vi "updated_hai-1.vi"() -> ()   [LabVIEW 2023]
uses:
  <vilib>/Utility/NIReport.llb/Report Type.ctl
  <vilib>/Utility/NIReport.llb/Append Text Table to Report (wrap).vi
  <vilib>/Utility/NIReport.llb/NI_report.lvclass
  <vilib>/Utility/NIReport.llb/NI_ReportGenerationCore.lvlib
  <vilib>/Utility/NIReport.llb/Excel/NI_Excel.lvclass
panel:
  out "Remaining_hours(hrs)":dbl
  out "Current flow out rate":dbl
  out "Current flow in rate":dbl
  out "Current water level  in litres:":dbl
  in  "Flow out rate(litres/sec)":dbl(slide) scale=0.0..10.0
  in  "Flow in rate(liters/sec)":dbl(slide) step=1.0 scale=0.0..10.0
  out "Water level is low":bool
  out "Water level is high":bool
  out "Tank":dbl(slide) scale=0.0..100.0
  in  "stop":bool
  in  "report file path":path
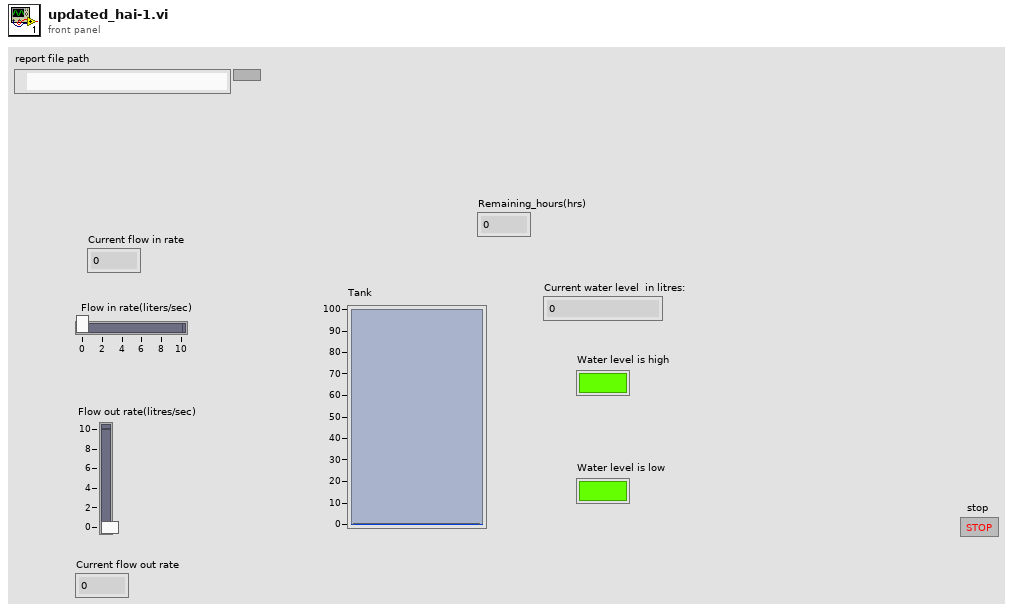
[diagram p1: front panel]
types:
  T1 = typedef "NI_ReportGenerationCore.lvlib/Report Type.ctl" = enum16{"HTML", "Word", "Excel"}
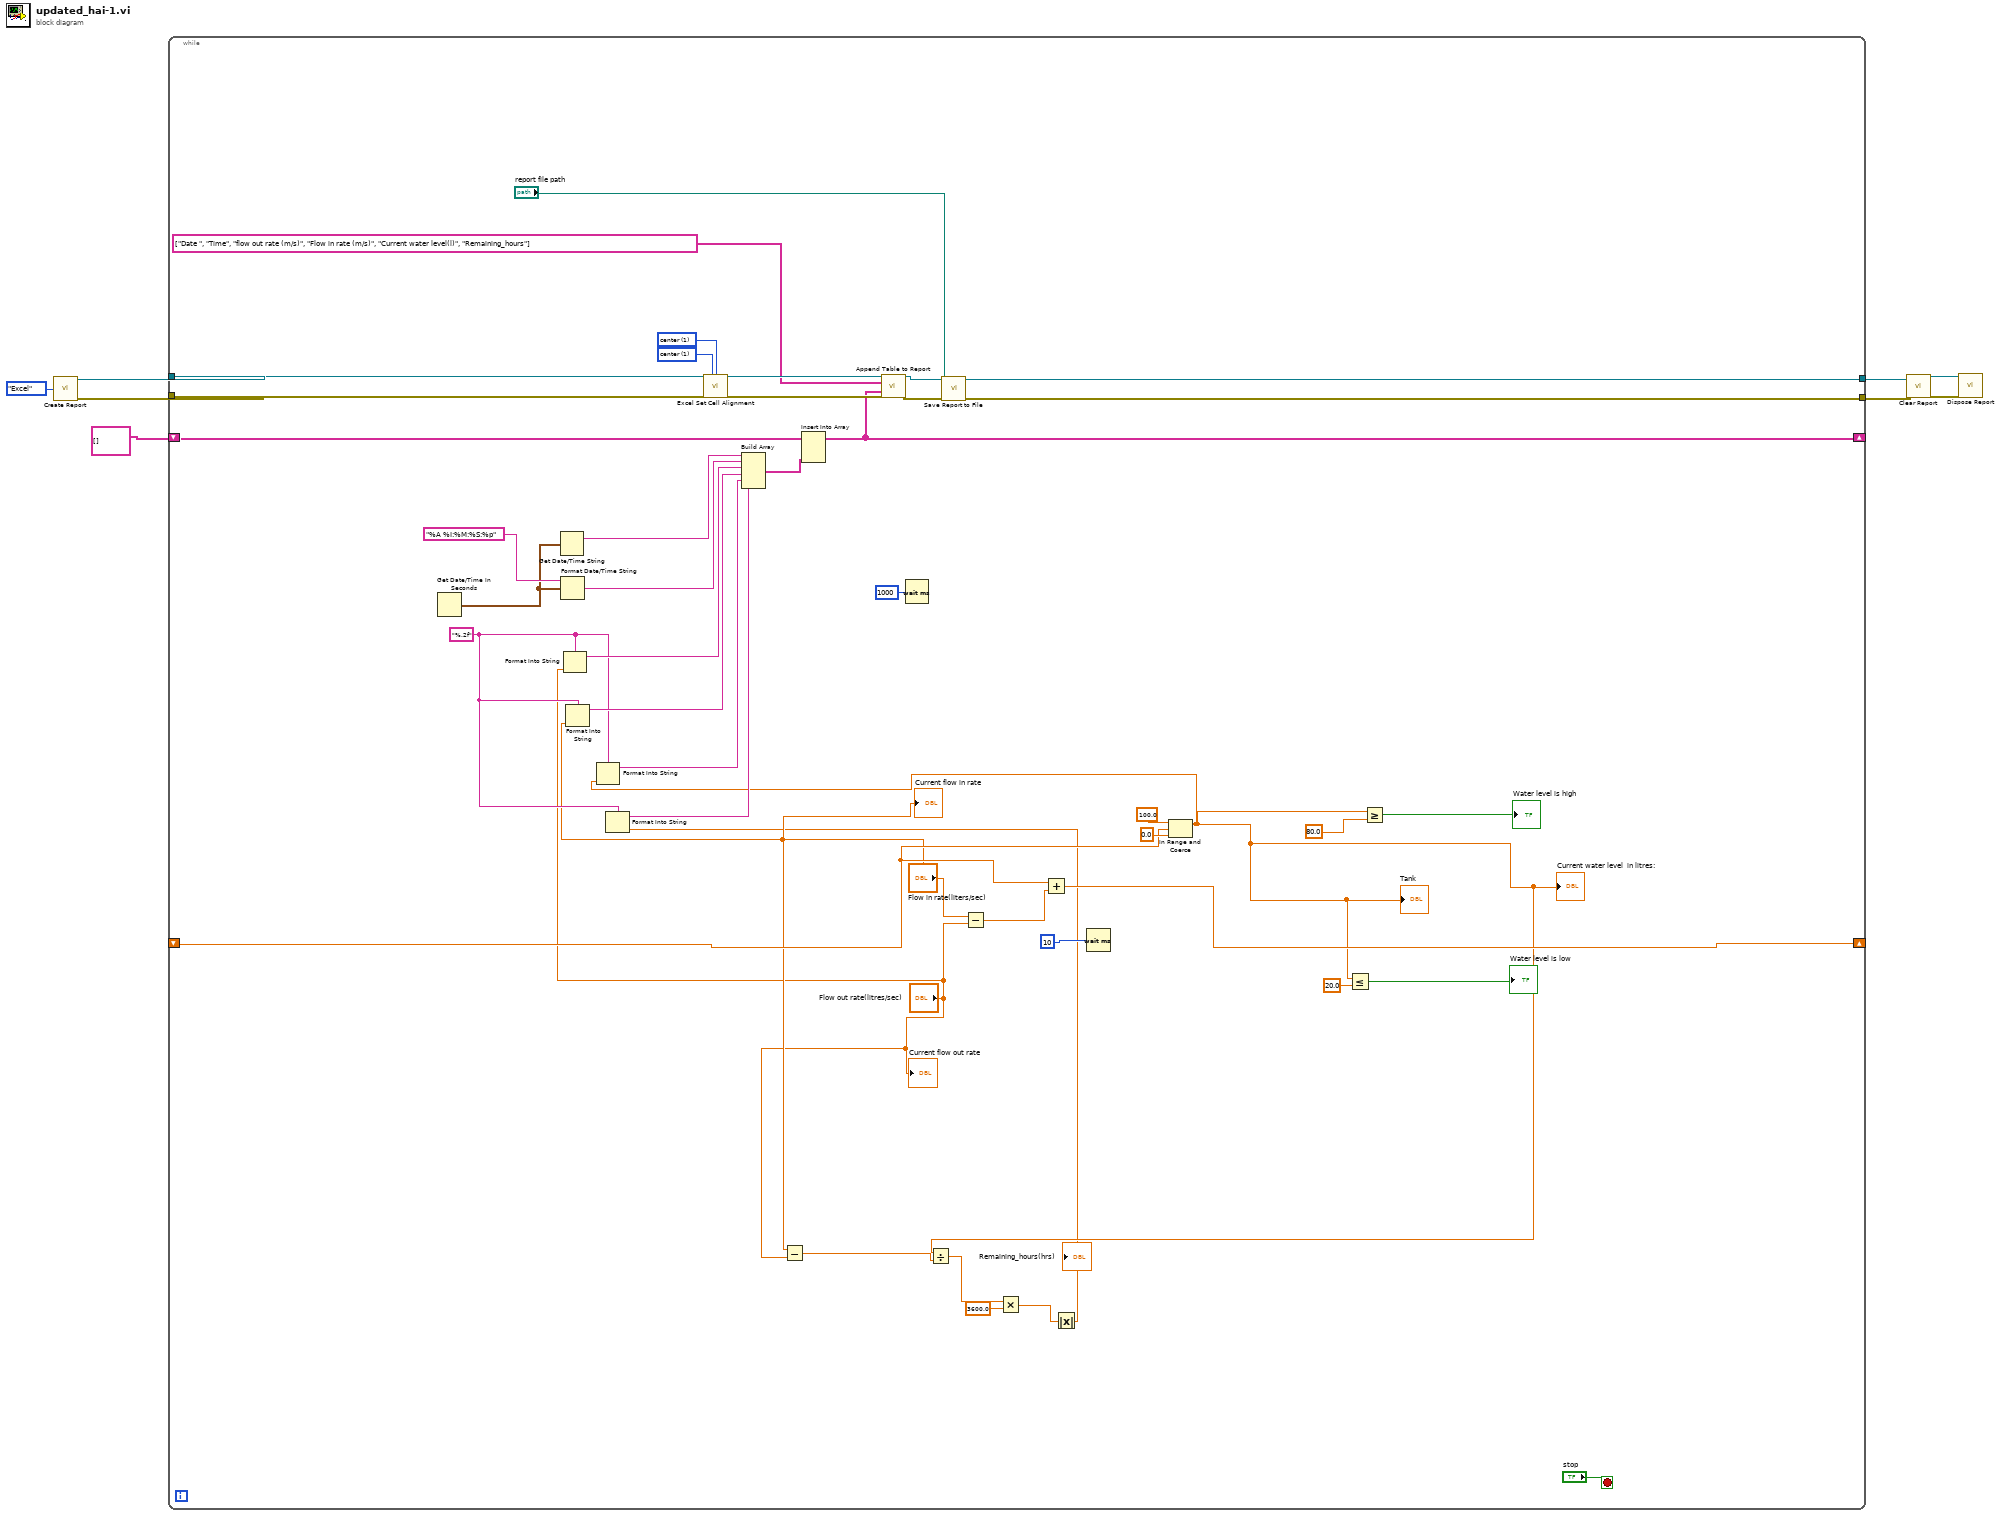
[diagram p0: block diagram]
diagram:
  n1 = call <vilib>:"Create Report.vi"("report type"=Report_Type."Excel") -> ("report out"=w7:refnum<class "NI_report.lvclass">, "error out"=w6:errorcluster)  [unwired: 13 in]
  n2 = while {
    tunnel: w7 -> [w52]
    tunnel: w6 -> [w51]
    tunnel: [w44] -> w5
    tunnel: [w43] -> w4
    shift-right: [w34] -> _
    shift-left: string[][] [] -> [w35]
    shift-right: [w21] -> _
    shift-left: _ -> [w20]
    stop <- "stop" stop-if-true
    w17 = "%.2f" ("format string")
    w49 = 1 items=["left", "center", "right"] ("horizontal alignment (left)")
    w50 = 1 items=["top", "center", "bottom"] ("vertical alignment (top)")
    n3 = Get Date/Time In Seconds() -> (seconds since 1Jan1904=w41:timestamp)
    n4 = Get Date/Time String(seconds (now)=w41) -> (date string=w40:string)  [unwired: 2 in, 1 out]
    n5 = Format Date/Time String(time format string (%c)="%A %I:%M:%S:%p", seconds (now)=w41) -> (date/time string=w39:string)  [unwired: 1 in]
    n6 = Format Into String(format string=w17, "Flow out rate(litres/sec)") -> (resulting string=w38:string)  [unwired: 2 in, 1 out]
    n7 = Format Into String(format string=w17, "Flow in rate(liters/sec)") -> (resulting string=w37:string)  [unwired: 2 in, 1 out]
    n8 = call <vilib>:"Excel Set Cell Alignment.vi"("report in"=w52, "vertical alignment (top)"=w50, "horizontal alignment (left)"=w49, "error in (no error)"=w51) -> ("report out"=w48:refnum<class "NI_report.lvclass">, "error out"=w47:errorcluster)  [unwired: 10 in]
    n9 = Subtract(x="Flow in rate(liters/sec)", y="Flow out rate(litres/sec)") -> (x-y=w13:dbl)
    n10 = Wait (ms)(milliseconds to wait=u32 1000) -> ()  [unwired: 1 out]
    n11 = Subtract(x="Flow in rate(liters/sec)", y="Flow out rate(litres/sec)") -> (x-y=w29:dbl)
    n12 = Add(x=w20, y=w29) -> (x+y=w21:dbl)
    n13 = Wait (ms)(milliseconds to wait=u32 10) -> ()  [unwired: 1 out]
    n14 = In Range and Coerce(upper limit=100.0, x=w20, lower limit=0.0) -> (coerced(x)=w14:dbl)  [unwired: 1 out]
    "Tank" <- w14
    "Current water level  in litres:" <- w14
    n15 = Format Into String(format string=w17, w14) -> (resulting string=w19:string)  [unwired: 2 in, 1 out]
    n16 = Divide(x=w14, y=w13) -> (x/y=w12:dbl)
    n17 = Multiply(x=w12, y=3600.0) -> (x*y=w10:dbl)
    n18 = Absolute Value(x=w10) -> (abs(x)=w9:dbl)
    "Remaining_hours(hrs)" <- w9
    n19 = Format Into String(format string=w17, w9) -> (resulting string=w18:string)  [unwired: 2 in, 1 out]
    n20 = Build Array(w40, w39, w38, w37, w19, w18) -> (w36:string[])
    n21 = Insert Into Array(array=w35, new element=w36) -> (w34:string[][])  [unwired: 2 in]
    n22 = call-poly <vilib>:"Append Table to Report.vi"("report in"=w48, "column headers"=string[] ["Date ", "Time", "flow out rate (m/s)", "Flow in rate (m/s)", "Current water level(l)", "Remaining_hours"] ("row headers"), "text data"=w34, "error in (no error)"=w47) -> ("report out"=w46:refnum<class "NI_report.lvclass">, "error out"=w45:errorcluster)  [unwired: 8 in, 2 out]
    n23 = call-dynamic "Save Report to File.vi"("report in"=w46, "report file path"="report file path", "error in (no error)"=w45) -> ("report out"=w44:refnum<class "NI_report.lvclass">, "error out"=w43:errorcluster)  [unwired: 11 in]
    n24 = Less Or Equal?(x=w14, y=20.0) -> (x <= y?=→"Water level is low":bool)
    n25 = Greater Or Equal?(x=w14, y=80.0) -> (x >= y?=→"Water level is high":bool)
    "Current flow in rate" <- "Flow in rate(liters/sec)"
    "Current flow out rate" <- "Flow out rate(litres/sec)"
  }
  n26 = call-dynamic "Clear Report.vi"("report in"=w5, "error in (no error)"=w4) -> ("report out"=w3:refnum<class "NI_report.lvclass">, "error out"=w2:errorcluster)  [unwired: 12 in]
  n27 = call-dynamic "Dispose Report.vi"("report in"=w3, "error in (no error)"=w2) -> ()  [unwired: 13 in, 1 out]
